vi "Close.vi"(8 "error in (no error)":errorcluster, 11 "Carya Config in":refnum<class "Carya Config (By Reference).lvclass">) -> (0 "error out":errorcluster)   [LabVIEW 2013, in "Carya Config (By Reference).lvclass"]
doc: "Copyright 2018, Carya Automatisering, Wiebe Walstra."
uses:
  Carya Config (By Reference).lvclass
  Carya Config (By Reference).lvclass/Carya Config (By Reference).ctl
  CConfig Buffer Type/CConfig Buffer Type.lvclass
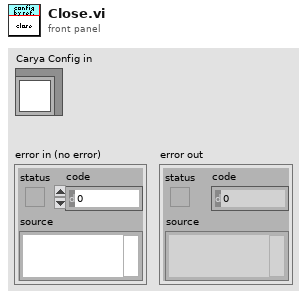
[diagram p1: front panel]
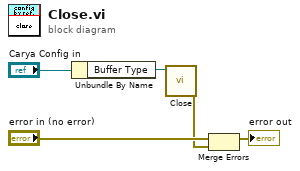
[diagram p0: block diagram]
diagram:
  n1 = Unbundle By Name("Carya Config in") -> ("Buffer Type"=w3:refnum<class "CConfig Buffer Type.lvclass">)
  n2 = call-dynamic "Close.vi"("Carya Config (Buffer) in"=w3) -> ("error out"=w1:errorcluster)  [unwired: 10 in]
  n3 = Merge Errors("error in (no error)", w1) -> (→"error out":errorcluster)
